vi "Filter Hold Data.vi"(10 "Data":dbl[][](array[numeric])) -> (1 "Mixed Mode Data":T1[](array[typedef]))   [LabVIEW 2013]
uses:
  Control Loop/Mixed Mode Hold Data type.ctl
  W:/NSEL OM/lib/Global Data/Names/Source Group Type.ctl
  Offsets Widget/Cartesian Or Actuator.ctl
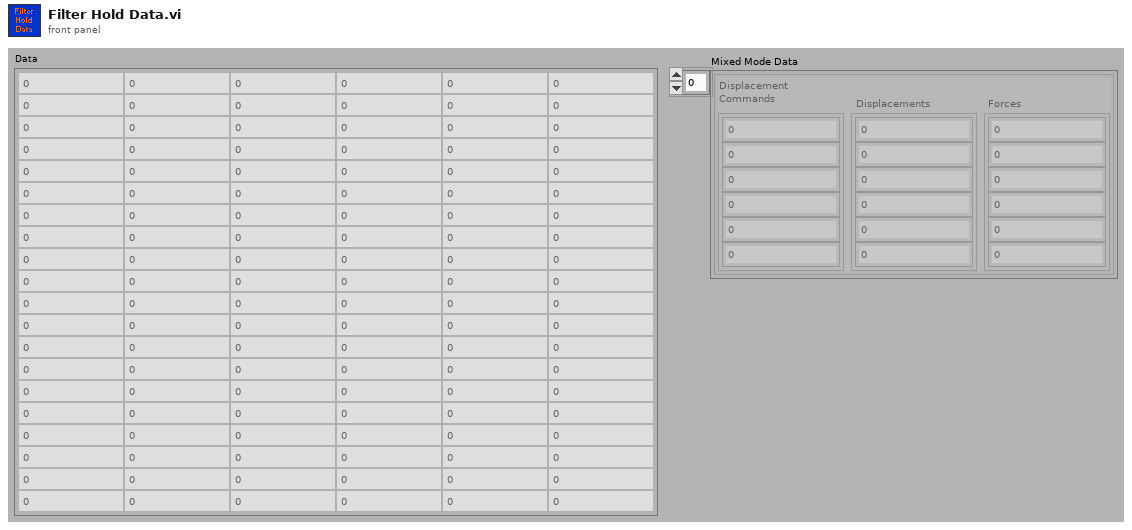
[diagram p1: front panel]
types:
  T1 = typedef "Mixed Mode Hold Data type.ctl" = cluster{"Displacements":dbl[], "Forces":dbl[], "Displacement \nCommands":dbl[]}
  T2 = typedef "Source Group Type.ctl" = enum16{"LBCB1", "LBCB2", "Consolidated", "External"}
  T3 = typedef "Cartesian Or Actuator.ctl" = bool
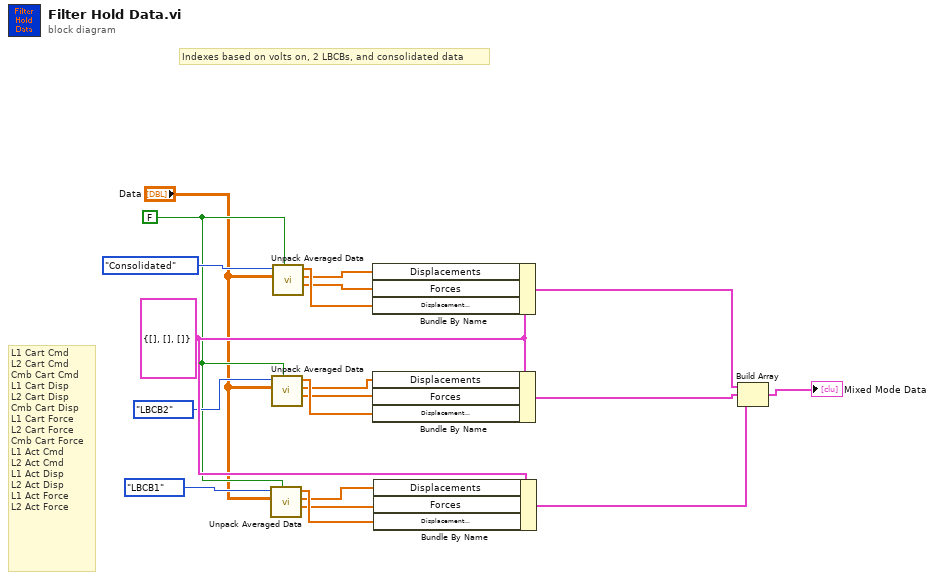
[diagram p0: block diagram]
diagram:
  w5 = T3 FALSE ("Coordinate Space")
  w16 = T1 {"Displacements"=[], "Forces"=[], "Displacement \nCommands"=[]} ("element")
  # "L1 Cart Cmd\nL2 Cart Cmd\nCmb Cart Cmd\nL1 Cart Disp\nL2 Cart Disp\nCmb Cart Disp\nL1 Cart Force\nL2 Cart Force\nCmb Cart Force\nL1 Act Cmd\nL2 Act Cmd\nL1 Act Disp\nL2 Act Disp \nL1 Act Force\nL2 Act Force"
  # "Indexes based on volts on, 2 LBCBs, and consolidated data"
  n1 = call "Unpack Averaged Data.vi"("Coordinate Space"=w5, "Data"="Data", "Source Group"=Source_Group_Type."LBCB1") -> ("Forces"=w1:dbl[], "Disp"=w2:dbl[], "Cmds"=w3:dbl[])  [unwired: 6 in]
  n2 = call "Unpack Averaged Data.vi"("Coordinate Space"=w5, "Data"="Data", "Source Group"=Source_Group_Type."LBCB2") -> ("Forces"=w7:dbl[], "Disp"=w8:dbl[], "Cmds"=w9:dbl[])  [unwired: 6 in]
  n3 = call "Unpack Averaged Data.vi"("Coordinate Space"=w5, "Data"="Data", "Source Group"=Source_Group_Type."Consolidated") -> ("Forces"=w11:dbl[], "Disp"=w12:dbl[], "Cmds"=w13:dbl[])  [unwired: 6 in]
  n4 = Bundle By Name(cluster=w16, "Displacements"=w12, "Forces"=w11, "Displacement \nCommands"=w13) -> (w19:T1)
  n5 = Bundle By Name(cluster=w16, "Displacements"=w8, "Forces"=w7, "Displacement \nCommands"=w9) -> (w18:T1)
  n6 = Bundle By Name(cluster=w16, "Displacements"=w2, "Forces"=w1, "Displacement \nCommands"=w3) -> (w15:T1)
  n7 = Build Array(w19, w18, w15) -> (→"Mixed Mode Data":T1[])
